vi "Sensor Readings.vi"() -> ()   [LabVIEW 2018]
panel:
  out "LimeLight_Valid":bool
  out "Battery_Voltage (V)":dbl
  out "Cargo_Captured":bool
  out "Hatch_Captured":bool
  in  "Range_Color_Front-Left":u32(colorbox)
  in  "Range_Color_Front-Right":u32(colorbox)
  in  "Range_Color_Left":u32(colorbox)
  in  "Range_Color_Right":u32(colorbox)
  in  "Range_Color_Rear":u32(colorbox)
  out "Front-Left_Prox_Sensor_(in)":dbl
  out "Front-Right_Prox_Sensor_(in)":dbl
  out "Rear_Prox_Sensor_(in)":dbl
  out "Left_Prox_Sensor_(in)":dbl
  out "Right_Prox_Sensor_(in)":dbl
  out "Ground_Sensor_(in)":dbl
  out "Tank_Pressure_(PSI)":dbl
  out "Lower_Intake_Current_(A)":dbl
  out "Upper_Intake_Current_(A)":dbl
  out "EncoderVel_Elevator":dbl
  out "EncoderPos_Elevator":dbl
  out "EncoderPos_Right_Drive":dbl
  out "EncoderPos_Left_Drive":dbl
  out "EncoderVel_Right_Drive":dbl
  out "EncoderVel_Left_Drive":dbl
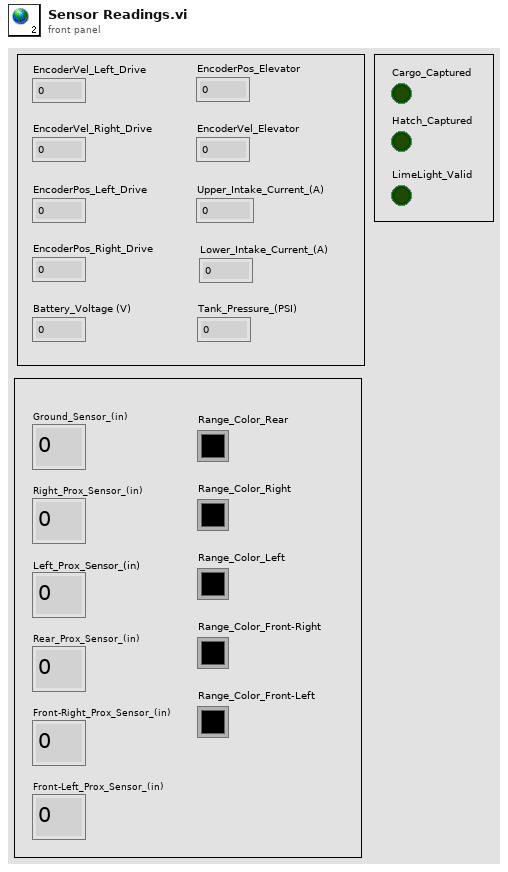
[diagram p1: front panel]
diagram:
